vi "State Change.vi"(10 "Self Actor State Transition":refnum<class "Self Actor State.lvclass">, 11 "Self Actor State Current":refnum<class "Self Actor State.lvclass">) -> (2 "Self Actor State out":refnum<class "Self Actor State.lvclass">)   [LabVIEW 2021, in "LVCAM.lvlib" / "Self Actor State.lvclass"]
uses:
  Self Actor State.lvclass
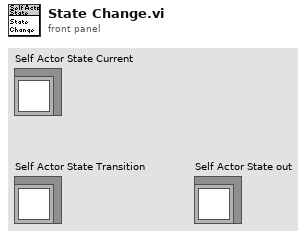
[diagram p1: front panel]
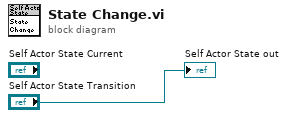
[diagram p0: block diagram]
diagram:
  "Self Actor State out" <- "Self Actor State Transition"
